vi "Shutdown Boiler.vi"(7 "MHL Queue in":refnum<queue>, 8 "error in":errorcluster, 9 "UI Data in":T1, 10 "Handshake Notifier in":refnum<notifier>, 11 "Boiler Queue in":refnum<queue>) -> (0 "error out":errorcluster, 1 "UI Data out":T1, 2 "Handshake Notifier out":refnum<notifier>, 3 "Boiler Queue out":refnum<queue>, 5 "MHL Queue out":refnum<queue>)   [LabVIEW 2017, in "Controller.lvlib"]
doc: "Shut down the boiler."
uses:
  Controller.lvlib
  support/Message Queue/Message Cluster.ctl
  controls/MHL UI Data.ctl
  controls/MHL Status.ctl
  support/Boiler System Globals.vi
  support/Message Queue/Message Queue.lvlib
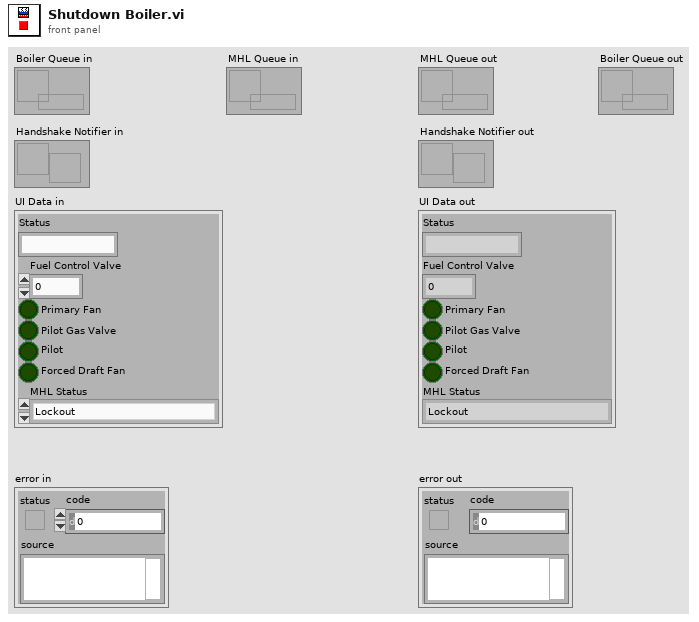
[diagram p1: front panel]
types:
  T1 = typedef "MHL UI Data.ctl" = cluster{"Status":string, "Fuel Control Valve":u32, "Primary Fan":bool, "Pilot Gas Valve":bool, "Pilot":bool, "Forced Draft Fan":bool, "MHL Status":T2}
  T2 = typedef "MHL Status.ctl" = enum16{"Lockout", "Ready", "Pre-Purge", "Pre-Purge Complete", "Pilot On", "Boiler Running", "Shutdown", "Purge"}
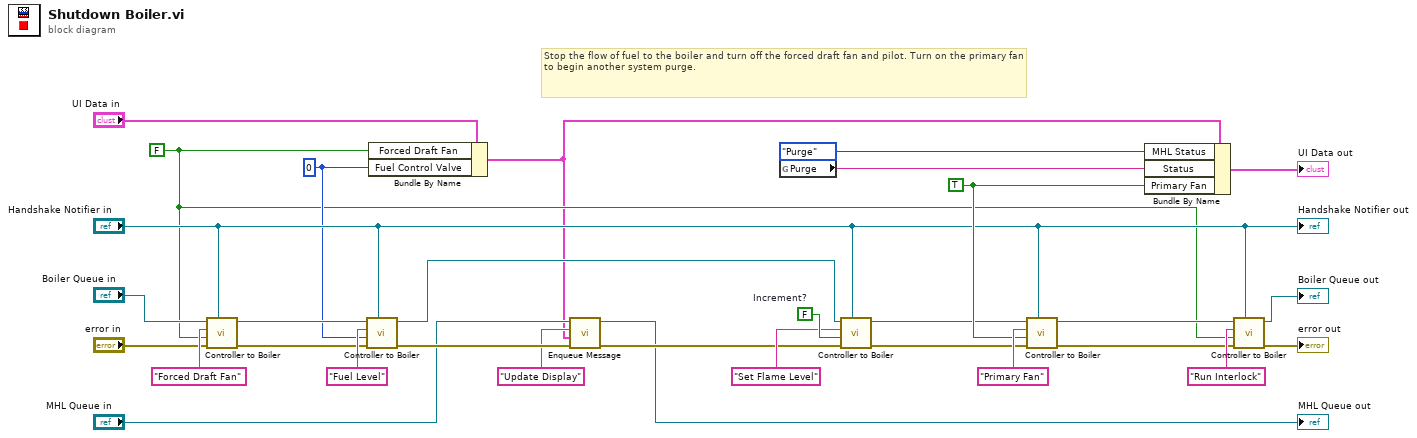
[diagram p0: block diagram]
diagram:
  w4 = u32 0 ("Fuel Control Valve Position Value")
  w3 = FALSE ("Fuel Valve")
  w22 = TRUE ("Primary Fan")
  w28 = FALSE  # Increment?
  # "Stop the flow of fuel to the boiler and turn off the forced draft fan and pilot. Turn on the primary fan to begin another system purge."
  n1 = call "Controller to Boiler.vi"("Notifier"="Handshake Notifier in", "error in"="error in", "Message Data"=w3, "Message"="Forced Draft Fan", "Boiler Queue in"="Boiler Queue in") -> ("error out"=w14:errorcluster, "Queue out"=w11:refnum<queue>)  [unwired: 4 in, 1 out]
  n2 = call "Controller to Boiler.vi"("Notifier"="Handshake Notifier in", "error in"=w14, "Message Data"=w4, "Message"="Fuel Level", "Boiler Queue in"=w11) -> ("error out"=w13:errorcluster, "Queue out"=w12:refnum<queue>)  [unwired: 4 in, 1 out]
  n3 = Bundle By Name(cluster="UI Data in", "Forced Draft Fan"=w3, "Fuel Control Valve"=w4) -> (w2:T1)
  n4 = call "Enqueue Message.vi"("error in (no error)"=w13, "Message Data"=w2, "Message"="Update Display", "Message Queue"="MHL Queue in") -> ("error out"=w8:errorcluster, "dup Message Queue"=→"MHL Queue out":refnum<queue>)  [unwired: 6 in]
  n5 = global read "Boiler System Globals.vi" "Purge"() -> (w20:string)
  n6 = call "Controller to Boiler.vi"("Notifier"="Handshake Notifier in", "error in"=w8, "Message Data"=w28, "Message"="Set Flame Level", "Boiler Queue in"=w12) -> ("error out"=w10:errorcluster, "Queue out"=w9:refnum<queue>)  [unwired: 4 in, 1 out]
  n7 = call "Controller to Boiler.vi"("Notifier"="Handshake Notifier in", "error in"=w10, "Message Data"=w22, "Message"="Primary Fan", "Boiler Queue in"=w9) -> ("error out"=w24:errorcluster, "Queue out"=w23:refnum<queue>)  [unwired: 4 in, 1 out]
  n8 = Bundle By Name(cluster=w2, "MHL Status"=MHL_Status."Purge", "Status"=w20, "Primary Fan"=w22) -> (→"UI Data out":T1)
  n9 = call "Controller to Boiler.vi"("Notifier"="Handshake Notifier in", "error in"=w24, "Message Data"=w3, "Message"="Run Interlock", "Boiler Queue in"=w23) -> ("error out"=→"error out":errorcluster, "Queue out"=→"Boiler Queue out":refnum<queue>)  [unwired: 4 in, 1 out]
  "Handshake Notifier out" <- "Handshake Notifier in"
